vi "TimedLoop-with-subvi-slot.vi"() -> ()   [LabVIEW 2026]
doc: "This VI illustrates how to use the Stop Timed Structure VI to programmatically abort a Timed Loop."
uses:
  <vilib>/Platform/TimedLoop/XDataNode/nitl_modes.ctl
  <vilib>/Platform/TimedLoop/XDataNode/timing_clust.ctl
  <vilib>/Platform/TimedLoop/XDataNode/wakeup.ctl
  <vilib>/platform/TimedLoop/XDataNode/XDataNode.xnode
  <vilib>/Platform/TimedLoop/XDataNode/XDNodeRunTimeDep.lvlib
panel:
  in  "stop":bool
  out "message":string
  in  "Abort":bool
  out "Current Iteration":i32
  # "Overview: Demonstrates the use of the Stop Timed Structure VI to programmatically abort a Timed Loop.\nRequirements: Windows\nInstructions:\n1. Run the VI.\n2. Click the Abort Timed Loop button. A dialog will indicate that the Timed Loop was programmatically aborted."
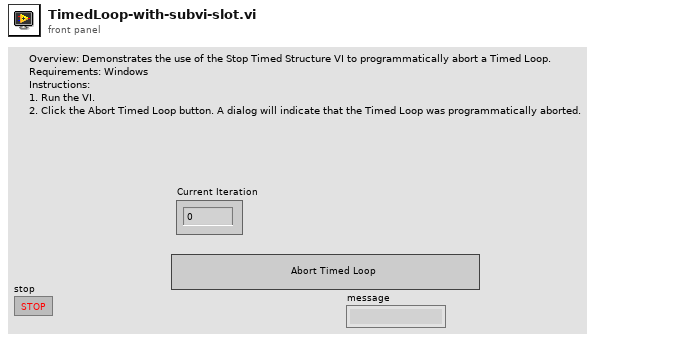
[diagram p1: front panel]
types:
  T1 = typedef "XDNodeRunTimeDep.lvlib/nitl_modes.ctl" = enum32{"No Change", "Process missed periods, maintain original phase", "Discard missed periods, maintain original phase", "Process missed periods, ignore original phase", "Discard missed periods, ignore original phase"}
  T2 = typedef "XDNodeRunTimeDep.lvlib/timing_clust.ctl" = cluster{"Expected End [f-1]":u64, "Actual End [f-1]":u64, "Finished Late? [f-1]":bool, "Expected End [i-1]":u64, "Actual End [i-1]":u64, "Finished Late? [i-1]":bool, "Expected Start [i]":u64, "Actual Start [i]":u64, "Expected Start [f]":u64, "Actual Start [f]":u64, "Source Name":string, "Structure Name":string, "Period":i64, "Deadline":i64, "Offset":i64, "Start":i64, "Priority":i32, "Timeout":i32, "Mode":T1, "Wakeup Reason":T3, "Error":errorcluster, "Source Type":string, "Secondary Source Type":string, "Global End Time":u64, "Global Start Time":u64, "Frame Duration":u64, "Iteration Duration":u64, "Assigned CPU":i32, "I/O Scan Engine Mode":u32}
  T3 = typedef "XDNodeRunTimeDep.lvlib/wakeup.ctl" = enum32{"Normal", "Aborted", "Asynchronous wakeup", "Timing source error", "Timed loop error", "Timeout"}
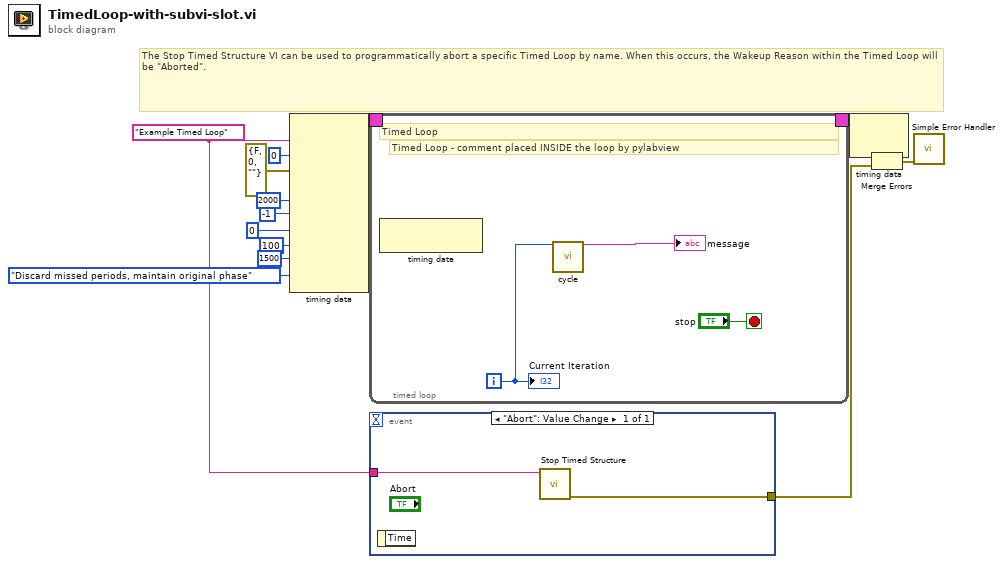
[diagram p0: block diagram]
diagram:
  w14 = "Example Timed Loop" ("Structure Name")
  # "The Stop Timed Structure VI can be used to programmatically abort a specific Timed Loop by name. When this occurs, the Wakeup Reason within the Timed Loop will be \"Aborted\"."
  n1 = node-c288(w14, 0 ("Processor"), errorcluster {"status"=FALSE, "code"=0, "source"=""} ("Error"), i64 2000 ("Period"), i64 -1 ("Deadline"), i64 0 ("Offset"), 100 ("Priority"), 1500 ("Timeout"), nitl_modes."Discard missed periods, maintain original phase" ("Mode")) -> (w12:T2)  [unwired: 1 in]
  n2 = timed-loop {
    timing: w12 -> [_]
    timing-out: [_] -> w13
    i -> [w17]
    stop <- "stop" stop-if-true
    # "Timed Loop - comment placed INSIDE the loop by pylabview"
    # "Timed Loop"
    n3 = node-c288() -> ()  [unwired: 1 in, 1 out]
    n4 = call "cycle.vi"("iteration"=w17) -> ("message"=→"message":string)  [unwired: 14 in]
    "Current Iteration" <- w17
  }
  n5 = event shown="[0] \"Abort\": Value Change" {
    selector: _ -> [_]
    dyn-events: _ -> [_]
    timeout: _ -> [_]
    tunnel: w14 -> [w21]
    tunnel: [w20] -> w10
    event "Abort": Value Change {
      n6 = event-data() -> ()  [unwired: 1 in, 1 out]
      n7 = call <vilib>:"Stop Timed Structure.vi"("name"=w21) -> ("error out"=w20:errorcluster)  [unwired: 10 in]
    }
  }
  n8 = node-c288(w13) -> (w11:errorcluster)
  n9 = Merge Errors(w11, w10) -> (w9:errorcluster)
  n10 = call <vilib>:"Simple Error Handler.vi"("error in (no error)"=w9) -> ()  [unwired: 4 in, 5 out]
